vi "SingleLoopTemplate.GetBroadcasts.vi"(11 "NewTemplate in":refnum<class "ErrorViewer.lvclass">) -> (2 "SingleLoopTemplate":cluster{"Broadcasts":T1, "Broadcasts":T2}, 3 "NewTemplate out":refnum<class "ErrorViewer.lvclass">)   [LabVIEW 2025, in "ErrorViewer.lvclass"]
uses:
  ErrorViewer.lvclass
  RQMHCore/ModuleCore/StandardBroadcasts.ctl
  RQMHCore/Shared/Died.ctl
  RQMHCore/ModuleCore/Started.ctl
  Broadcast Events--cluster.ctl
  Stopped.ctl
  RQMHCore/ModuleCore/RQMHModule.lvclass/RQMHModule.ctl
  ErrorViewer.lvclass/ErrorViewer.ctl
  C:/Git/JA/JQMH/RQMHCore/ModuleCore/RQMHModule.lvclass
  C:/Git/JA/JQMH/ModuleTemplates/ErrorViewer/ErrorViewer.lvclass
  RQMHCore/ModuleCore/RQMHModule.lvclass
  RQMHCore/Shared/RQMHShared.lvlib
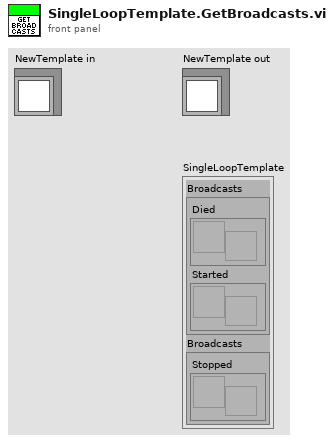
[diagram p1: front panel]
types:
  T1 = typedef "RQMHModule.lvclass/StandardBroadcasts.ctl" = cluster{"Died":refnum<user-event>, "Started":refnum<user-event>}
  T2 = typedef "ErrorViewer.lvclass/Broadcast Events--cluster.ctl" = cluster{"Stopped":refnum<user-event>}
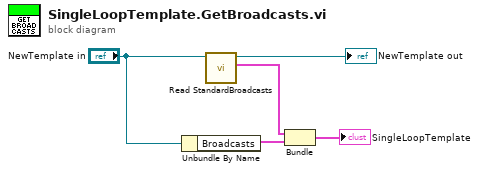
[diagram p0: block diagram]
diagram:
  n1 = Unbundle By Name("NewTemplate in") -> ("Broadcasts"=w5:T2)
  n2 = call "Read StandardBroadcasts.vi"("JQMHCore in"="NewTemplate in") -> ("Broadcasts"=w4:T1, "JQMHCore out"=→"NewTemplate out":refnum<class "ErrorViewer.lvclass">)  [unwired: 8 in, 1 out]
  n3 = Bundle("Broadcasts"=w4, "Broadcasts"=w5) -> (→"SingleLoopTemplate":cluster{"Broadcasts":T1, "Broadcasts":T2})  [unwired: 1 in]
